vi "pinv_error.vi"(2 "Y":sgl[][](array[numeric]), 4 "Calibrated":T1) -> (1 "Error":dbl)   [LabVIEW 2013]
uses:
  <vilib>/Analysis/Matrix/Datatypes/RealMatrix.ctl
  <vilib>/Analysis/Matrix/Numeric/Subtract/Subtract - RM,RM.vi
  <vilib>/Analysis/Matrix/NI_Matrix.lvlib
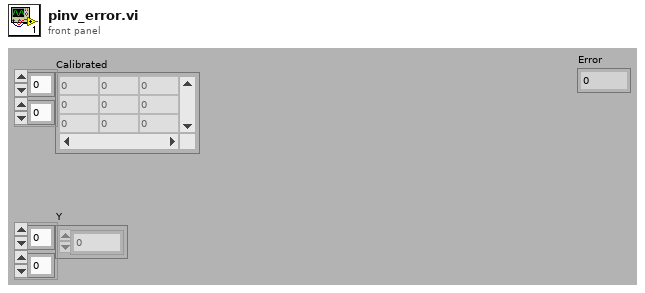
[diagram p1: front panel]
types:
  T1 = typedef "NI_Matrix.lvlib/RealMatrix.ctl" = dbl[][]
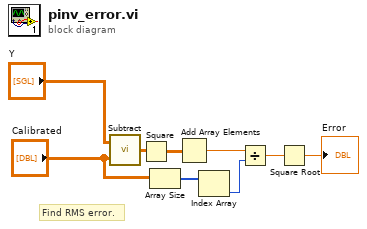
[diagram p0: block diagram]
diagram:
  # "Find RMS error."
  n1 = call-poly <vilib>:"Subtract.vi"("Real Matrix B"="Calibrated", "Real Matrix A"="Y") -> ("A - B"=w2:T1)
  n2 = Square(x=w2) -> (x^2=w3:T1)
  n3 = Array Size(array="Calibrated") -> (size(s)=w8:i32[])
  n4 = Add Array Elements(numeric array=w3) -> (sum=w4:dbl)
  n5 = Index Array(array=w8) -> (element=w9:i32)  [unwired: 1 in]
  n6 = Divide(x=w4, y=w9) -> (x/y=w6:dbl)
  n7 = Square Root(x=w6) -> (sqrt(x)=→"Error":dbl)
